vi "Periodic Tasks.vi"() -> ()   [LabVIEW 2014]
doc: "This VI runs in parallel to other tasks. It can contain as many user-defined periodic loops as you need. These can carry out PID or other sorts of timed response."
uses:
  <vilib>/Rock Robotics/WPI/DriverStation/WPI_DriverStationRobotMode2.ctl
  Global Variables.vi
  Robot Global Data.vi
  <vilib>/Utility/file.llb/Read From Spreadsheet File (DBL).vi
  <vilib>/Utility/file.llb/Write To Spreadsheet File (DBL).vi
  <vilib>/addons/control/pid/NI_PID_pid.lvlib
  <vilib>/addons/control/pid/pid.llb/PID (DBL).vi
  NavX Code/navX-MXP Library/navX-MXP IMU.lvlib
  <vilib>/Rock Robotics/WPI/DriverStation/WPI_DriverStationStatusErrorCache.ctl
panel:
  in  "Left Rumble":sgl
  in  "Right Rumble":sgl
  out "Degrees":u16
  out "navX Data":u8[](array[numeric])
  in  "PID gains":T1={"proportional gain (Kc)"=1.0, "integral time (Ti, min)"=0.01, "derivative time (Td, min)"=0.0} {"derivative time (Td, min)" format="%.3f"; "integral time (Ti, min)" format="%.3f"; "proportional gain (Kc)" format="%.3f"}
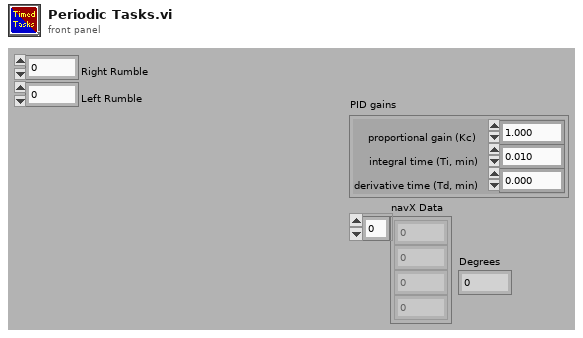
[diagram p1: front panel]
types:
  T1 = cluster{"proportional gain (Kc)":dbl, "integral time (Ti, min)":dbl, "derivative time (Td, min)":dbl}
  T2 = enum16{"Stop", "Three Tote", "Two Tote", "One Tote", "Step", "Top", "Home", "Joystick"}
  T3 = typedef "navX-MXP IMU.lvlib/navX Device TypeDef.ctl" = cluster{"navX Interface Protocol":T4, "navX Interface Protocol TypeDefs":cluster{"SPIDevRef":T5, "I2CDevRef":T8}, "navX System Information":cluster{"Board Information":T10, "Status":T11, "Offsets":T15}, "navX Common Information":cluster{"Update Rate (4Hz-60Hz)":T16, "refnum name":string, "error":errorcluster}}
  T4 = typedef "navX-MXP IMU.lvlib/navX Interface Protocol.ctl" = enum16{"SPI", "I2C"}
  T5 = typedef "WPI_SPIDevRef.ctl" = cluster{"DevStatus":errorcluster, "Handle":i32, "Controller":T6, "SPI Bus":T7}
  T6 = typedef "FPGA_TypedefDigitalModule.ctl" = enum16{"Controller 1"}
  T7 = typedef "spi_bus.ctl" = enum16{"SPI On-Board, CS0", "SPI On-Board, CS1", "SPI On-Board, CS2", "SPI On-Board, CS3", "SPI MXP", "Invalid"}
  T8 = typedef "WPI_I2CDevRef.ctl" = cluster{"DevStatus":errorcluster, "Controller":T6, "Device Address":u8, "Handle":i32, "I2C Bus":T9}
  T9 = typedef "i2c_bus.ctl" = enum16{"I2C On-Board", "I2C MXP", "Invalid"}
  T10 = typedef "navX-MXP IMU.lvlib/navX Board Information.ctl" = cluster{"WhoAmI (50 | 0x32)":u8, "Board Revision":u8, "Firmware Major Version":u8, "Firmware Minor Version":u8}
  T11 = typedef "navX-MXP IMU.lvlib/navX Status Data.ctl" = cluster{"Update Rate Hz":u8, "Accelerometer Full-Scale Range":u8, "Gyro Full-Scale Range":u16, "NAVX_OP_STATUS":T12, "NAVX_CAL_STATUS":T13, "NAVX_SELFTEST_STATUS":u8, "NAVX_SENSOR_STATUS":T14}
  T12 = typedef "navX-MXP IMU.lvlib/navX NAVX_OP_STATUS.ctl" = u8
  T13 = typedef "navX-MXP IMU.lvlib/navX NAVX_CAL_STATUS.ctl" = u8
  T14 = typedef "navX-MXP IMU.lvlib/navX NAVX_SENSOR_STATUS.ctl" = cluster{"MOVING":bool, "YAW_STABLE":bool, "MAG_DISTURBANCE":bool, "ALTITUDE_VALID":bool, "SEALEVEL_PRESS_SET":bool, "FUSED_HEADING_VALID":bool}
  T15 = typedef "navX-MXP IMU.lvlib/navX Offsets Data.ctl" = cluster{"Yaw":dbl, "Quat W":dbl, "Quat X":dbl, "Quat Y":dbl, "Quat Z":dbl}
  T16 = typedef "navX-MXP IMU.lvlib/navX Update Rate.ctl" = u8
  T17 = typedef "WPI_DriverStationStatusErrorCache.ctl" = enum16{"Get", "Set"}
  T18 = typedef "WPI_JoystickDevRef.ctl" = cluster{"Device":T19}
  T19 = typedef "WPI_JoystickDeviceEnum.ctl" = enum16{"USB 0", "USB 1", "USB 2", "USB 3", "USB 4", "USB 5"}
  T20 = typedef "WPI_MotorControlDeviceRef.ctl" = cluster{"DeviceStatus":errorcluster, "Type":T21, "PWM":cluster{"Controller":T6, "PWM Channel":T22, "DeadBand":T23}, "CAN":cluster{"Device Number":u8, "Control Mode":T24, "Semaphore":T25, "Max Vout":dbl, "TalonSRX Control Mode":T26}, "Invert":bool, "TransformRef":T27, "InvTransformRef":T27}
  T21 = typedef "WPI_MotorControlType.ctl" = enum16{"PWM", "CAN", "CANTalonSRX"}
  T22 = typedef "FPGA_DIOPWMChannel.ctl" = enum8{"PWM 0", "PWM 1", "PWM 2", "PWM 3", "PWM 4", "PWM 5", "PWM 6", "PWM 7", "PWM 8", "PWM 9", "PWM MXP 0", "PWM MXP 1", "PWM MXP 2", "PWM MXP 3", "PWM MXP 4", "PWM MXP 5", "PWM MXP 6", "PWM MXP 7", "PWM MXP 8", "PWM MXP 9", "Invalid"}
  T23 = typedef "WPI_PWMDeadband.ctl" = cluster{"Name":string, "maxPositivePwm":i32, "minPositivePwm":i32, "centerPwm":i32, "maxNegativePwm":i32, "minNegativePwm":i32, "angularRange":u16}
  T24 = typedef "WPI_CANJaguar_ControlMode.ctl" = enum8{"Percent VBus", "Current", "Speed", "Position", "Voltage"}
  T25 = typedef "Semaphore RefNum" = refnum<k1>
  T26 = typedef "WPI_CANTalonSRX_APIControlMode.ctl" = enum8{"Percent VBus", "Speed", "Position", "Slave", "Unchanged / Invalid"}
  T27 = typedef "WPI_PWMTransform_ConPane.ctl" = refnum<vi>
  T28 = typedef "WPI_DriverStationRobotMode2.ctl" = enum16{"Autonomous Disabled", "Autonomous Enabled", "Teleop Disabled", "Teleop Enabled", "Disconnected", "Finish", "Test Disabled", "Test Enabled", "Emergency Stopped"}
  T29 = typedef "WPI_CounterDevRef.ctl" = cluster{"DevStatus":errorcluster, "CntIndex":T30}
  T30 = typedef "FPGA_CounterCtrSystemIndex.ctl" = enum8{"Ctr 0", "Ctr 1", "Ctr 2", "Ctr 3", "Ctr 4", "Ctr 5", "Ctr 6", "Ctr 7", "Invalid"}
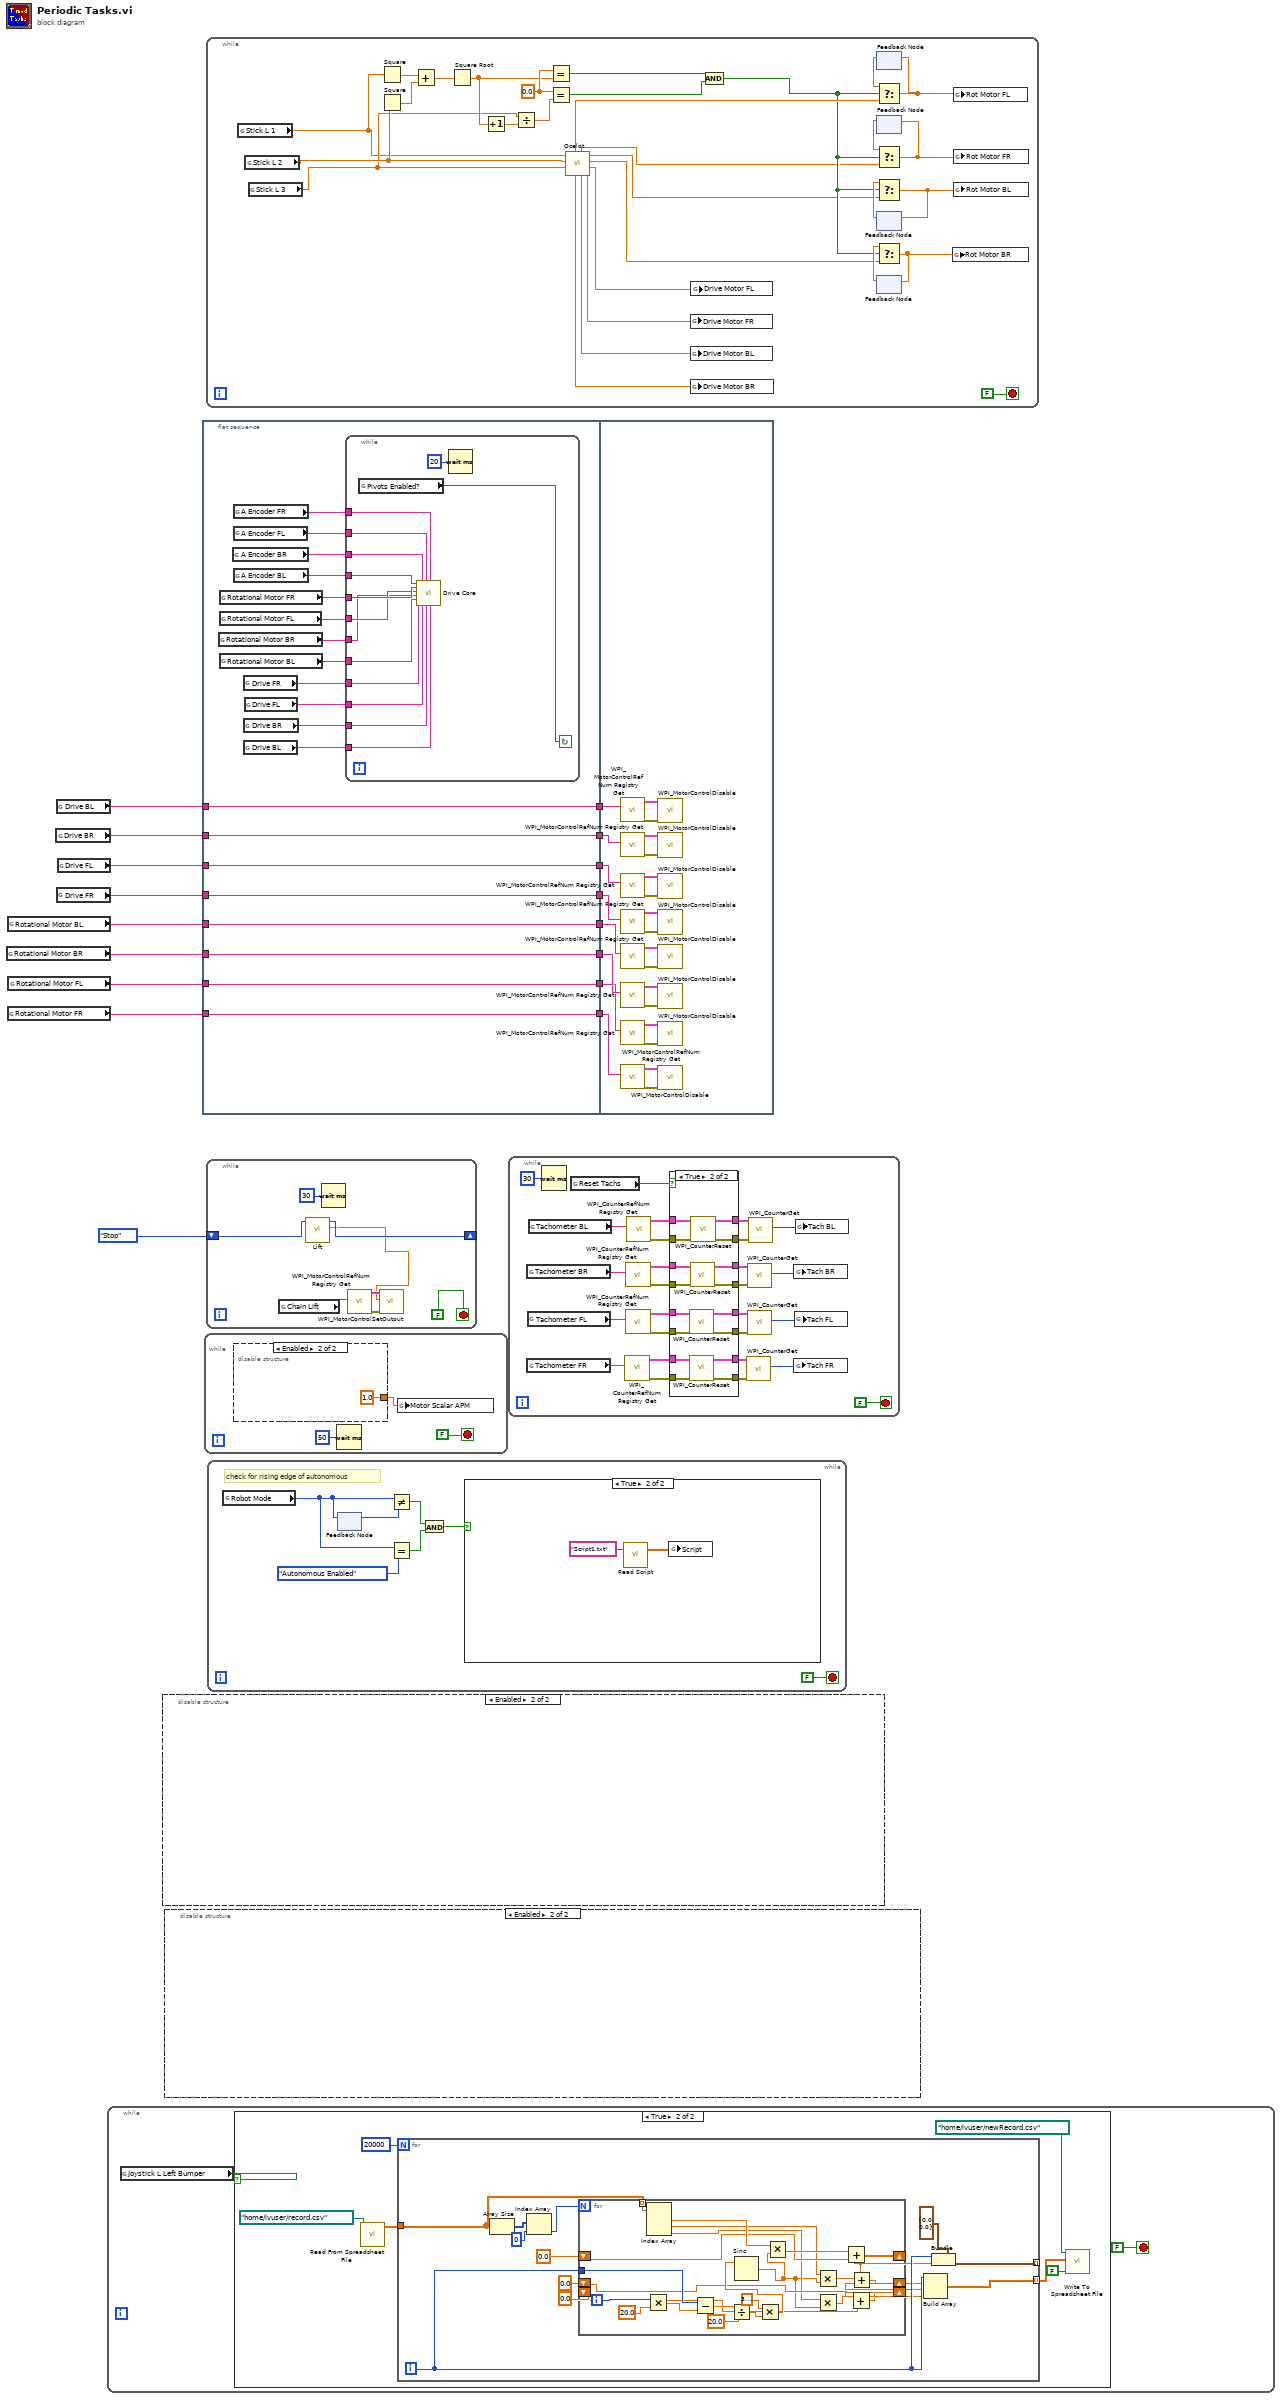
[diagram p0: block diagram]
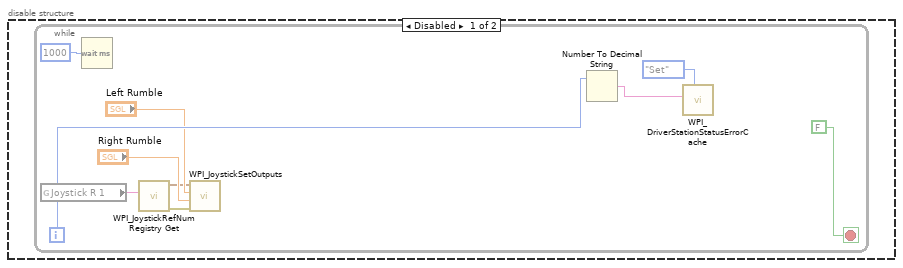
[diagram p3: hidden frame]
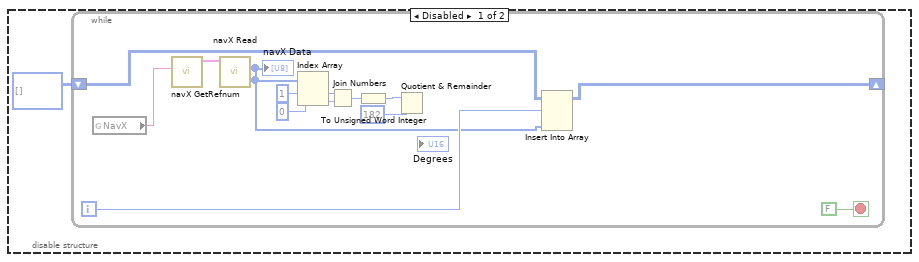
[diagram p4: hidden frame]
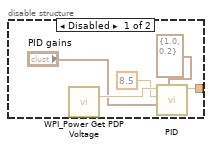
[diagram p7: hidden frame]
diagram:
  n1 = global read "Global Variables.vi" "Rotational Motor BR"() -> (w6:string)
  n2 = global read "Global Variables.vi" "Rotational Motor BL"() -> (w8:string)
  n3 = global read "Global Variables.vi" "Rotational Motor FR"() -> (w2:string)
  n4 = global read "Global Variables.vi" "Rotational Motor FL"() -> (w4:string)
  n5 = global read "Global Variables.vi" "Drive BR"() -> (w14:string)
  n6 = global read "Global Variables.vi" "Drive BL"() -> (w16:string)
  n7 = global read "Global Variables.vi" "Drive FR"() -> (w10:string)
  n8 = global read "Global Variables.vi" "Drive FL"() -> (w12:string)
  n9 = while {
    stop <- FALSE stop-if-true
    n10 = global read "Global Variables.vi" "Joystick L Left Bumper"() -> (w18:bool)
    n11 = case shown="True" w18 {
      frame False {
      }
      frame True {
        n12 = call-poly <vilib>:"Read From Spreadsheet File.vi"("file path (dialog if empty)"=path "/home/lvuser/record.csv") -> ("all rows"=w24:dbl[][])  [unwired: 6 in, 4 out]
        n13 = for {
          N: 20000 -> [_]
          tunnel: [w34] -> _ mode=indexing
          tunnel: w24 -> [w33]
          tunnel: [w30] -> w23 mode=indexing
          i -> [w32]
          n14 = Array Size(array=w33) -> (size(s)=w39:i32[])
          n15 = Index Array(array=w39, index=0) -> (element=w38:i32)
          n16 = for {
            N: w38 -> [_]
            shift-right: [w49] -> w31
            shift-left: 0.0 -> [w51]
            tunnel: w33 -> [w60] mode=indexing
            tunnel: w32 -> [w52]
            shift-right: [w47] -> w29
            shift-left: 0.0 -> [w44]
            shift-right: [w48] -> w28
            shift-left: 0.0 -> [w43]
            i -> [w58]
            n17 = Multiply(x=w58, y=20.0) -> (x*y=w55:dbl)
            n18 = Index Array(array=w60) -> (element #1=w61:dbl, element #2=w42:dbl, element #3=w41:dbl)  [unwired: 3 in]
            n19 = Subtract(x=w52, y=w55) -> (x-y=w57:dbl)
            n20 = Divide(x=w57, y=20.0) -> (x/y=w54:dbl)
            n21 = Multiply(x=3.141592653589793, y=w54) -> (x*y=w50:dbl)
            n22 = Sinc(1:w50) -> (0:w40:dbl)
            n23 = Multiply(x=w61, y=w40) -> (x*y=w62:dbl)
            n24 = Multiply(x=w42, y=w40) -> (x*y=w45:dbl)
            n25 = Multiply(x=w41, y=w40) -> (x*y=w46:dbl)
            n26 = Add(x=w62, y=w51) -> (x+y=w49:dbl)
            n27 = Add(x=w46, y=w43) -> (x+y=w48:dbl)
            n28 = Add(x=w45, y=w44) -> (x+y=w47:dbl)
          }
          n29 = Build Array(w32, w31, w29, w28) -> (w30:dbl[])
          n30 = Bundle(cluster=cluster{dbl, dbl} {0.0, 0.0}, w32, w31) -> (w34:cluster{dbl, dbl})
        }
        n31 = call-poly <vilib>:"Write To Spreadsheet File.vi"("append to file? (new file:F)"=FALSE, "2D data"=w23, "file path (dialog if empty)"=path "/home/lvuser/newRecord.csv") -> ()  [unwired: 5 in, 1 out]
      }
    }
  }
  n32 = disable-structure shown="Enabled" {
    frame Disabled {
      n33 = while {
        shift-right: [w66] -> _
        shift-left: u16[][] [] -> [w65]
        i -> [w67]
        stop <- FALSE stop-if-true
        n34 = global read "Global Variables.vi" "NavX"() -> (w75:string)
        n35 = call "navX GetRefnum.vi"("refnum name"=w75) -> ("navX Device TypeDef"=w76:T3)  [unwired: 9 in, 1 out]
        n36 = call "navX Read.vi"("navX Device TypeDef"=w76) -> ("navX Data"=w64:u8[])  [unwired: 8 in, 2 out]
        "navX Data" <- w64
        n37 = Index Array(array=w64, index #1=1 ("index"), index #2=0 ("index")) -> (element #1=w74:u8, element #2=w73:u8)
        n38 = Join Numbers(hi=w74, lo=w73) -> ((hi.lo)=w70:u16)
        n39 = To Unsigned Word Integer(number=w70) -> (unsigned 16bit integer=w69:u16)
        n40 = Quotient & Remainder(x=w69, y=u16 182) -> ()  [unwired: 2 out]
        n41 = Insert Into Array(array=w65, index (row)=w67, new element=w64) -> (w66:u16[][])  [unwired: 1 in]
      }
    }
    frame Enabled {
    }
  }
  n42 = disable-structure shown="Enabled" {
    frame Disabled {
      n43 = while {
        i -> [w84]
        stop <- FALSE stop-if-true
        n44 = global read "Global Variables.vi" "Joystick R 1"() -> (w79:string)
        n45 = Wait (ms)(milliseconds to wait=u32 1000) -> ()  [unwired: 1 out]
        n46 = call <vilib>:"WPI_JoystickRefNum Registry Get.vi"("refnum name"=w79) -> ("error out"=w78:errorcluster, "JoystickDevRef"=w80:T18)  [unwired: 9 in]
        n47 = call <vilib>:"WPI_JoystickSetOutputs.vi"("error in (no error)"=w78, "Right Rumble"="Right Rumble", "Left Rumble"="Left Rumble", "JoystickDevRef"=w80) -> ()  [unwired: 6 in, 2 out]
        n48 = Number To Decimal String(number=w84) -> (decimal integer string=w85:string)  [unwired: 1 in]
        n49 = call <vilib>:"WPI_DriverStationStatusErrorCache.vi"("StatusErrorCacheOp"=WPI_DriverStationStatusErrorCache."Set", "Error String"=w85) -> ()  [unwired: 1 in, 9 out]
      }
    }
    frame Enabled {
    }
  }
  n50 = flat-sequence {
    tunnel: [w95] -> w17
    tunnel: w16 -> [w95]
    tunnel: [w94] -> w15
    tunnel: w14 -> [w94]
    tunnel: [w93] -> w13
    tunnel: w12 -> [w93]
    tunnel: [w92] -> w11
    tunnel: w10 -> [w92]
    tunnel: [w91] -> w9
    tunnel: w8 -> [w91]
    tunnel: [w90] -> w7
    tunnel: w6 -> [w90]
    tunnel: [w89] -> w5
    tunnel: w4 -> [w89]
    tunnel: [w88] -> w3
    tunnel: w2 -> [w88]
    tunnel: w17 -> [w129]
    tunnel: w15 -> [w128]
    tunnel: w13 -> [w127]
    tunnel: w11 -> [w126]
    tunnel: w9 -> [w125]
    tunnel: w7 -> [w124]
    tunnel: w5 -> [w123]
    tunnel: w3 -> [w122]
    frame #0 {
      n51 = global read "Global Variables.vi" "Rotational Motor BR"() -> (w101:string)
      n52 = global read "Global Variables.vi" "Rotational Motor FR"() -> (w103:string)
      n53 = global read "Global Variables.vi" "Rotational Motor FL"() -> (w102:string)
      n54 = global read "Global Variables.vi" "Rotational Motor BL"() -> (w100:string)
      n55 = global read "Global Variables.vi" "A Encoder BR"() -> (w105:string)
      n56 = global read "Global Variables.vi" "A Encoder FR"() -> (w107:string)
      n57 = global read "Global Variables.vi" "A Encoder FL"() -> (w106:string)
      n58 = global read "Global Variables.vi" "A Encoder BL"() -> (w104:string)
      n59 = global read "Global Variables.vi" "Drive FR"() -> (w99:string)
      n60 = global read "Global Variables.vi" "Drive BR"() -> (w97:string)
      n61 = global read "Global Variables.vi" "Drive BL"() -> (w96:string)
      n62 = global read "Global Variables.vi" "Drive FL"() -> (w98:string)
      n63 = while {
        tunnel: w107 -> [w120]
        tunnel: w106 -> [w119]
        tunnel: w105 -> [w118]
        tunnel: w104 -> [w117]
        tunnel: w103 -> [w116]
        tunnel: w102 -> [w115]
        tunnel: w101 -> [w114]
        tunnel: w100 -> [w113]
        tunnel: w99 -> [w112]
        tunnel: w98 -> [w111]
        tunnel: w97 -> [w110]
        tunnel: w96 -> [w109]
        stop <- w121 continue-if-true
        n64 = global read "Global Variables.vi" "Pivots Enabled?"() -> (w121:bool)
        n65 = call "Drive Core.vi"("A Encoder BL"=w117, "Rotational Motor FR"=w116, "Rotational Motor FL"=w115, "Rotational Motor BR"=w114, "Rotational Motor BL"=w113, "Drive Motor FR"=w112, "A Encoder BR"=w118, "Drive Motor FL"=w111, "A Encoder FL"=w119, "Drive Motor BR"=w110, "A Encoder FR"=w120, "Drive Motor BL"=w109) -> ()  [unwired: 8 in]
        n66 = Wait (ms)(milliseconds to wait=u32 20) -> ()  [unwired: 1 out]
      }
    }
    frame #1 {
      n67 = call <vilib>:"WPI_MotorControlRefNum Registry Get.vi"("refnum name"=w129) -> ("error out"=w145:errorcluster, "MotorControlDevRef"=w144:T20)  [unwired: 9 in]
      n68 = call <vilib>:"WPI_MotorControlRefNum Registry Get.vi"("refnum name"=w128) -> ("error out"=w143:errorcluster, "MotorControlDevRef"=w142:T20)  [unwired: 9 in]
      n69 = call <vilib>:"WPI_MotorControlRefNum Registry Get.vi"("refnum name"=w127) -> ("error out"=w141:errorcluster, "MotorControlDevRef"=w140:T20)  [unwired: 9 in]
      n70 = call <vilib>:"WPI_MotorControlRefNum Registry Get.vi"("refnum name"=w126) -> ("error out"=w139:errorcluster, "MotorControlDevRef"=w138:T20)  [unwired: 9 in]
      n71 = call <vilib>:"WPI_MotorControlRefNum Registry Get.vi"("refnum name"=w125) -> ("error out"=w137:errorcluster, "MotorControlDevRef"=w136:T20)  [unwired: 9 in]
      n72 = call <vilib>:"WPI_MotorControlRefNum Registry Get.vi"("refnum name"=w124) -> ("error out"=w135:errorcluster, "MotorControlDevRef"=w134:T20)  [unwired: 9 in]
      n73 = call <vilib>:"WPI_MotorControlRefNum Registry Get.vi"("refnum name"=w123) -> ("error out"=w133:errorcluster, "MotorControlDevRef"=w132:T20)  [unwired: 9 in]
      n74 = call <vilib>:"WPI_MotorControlRefNum Registry Get.vi"("refnum name"=w122) -> ("error out"=w131:errorcluster, "MotorControlDevRef"=w130:T20)  [unwired: 9 in]
      n75 = call <vilib>:"WPI_MotorControlDisable.vi"("error in (no error)"=w145, "MotorControlDevRef"=w144) -> ()  [unwired: 8 in, 2 out]
      n76 = call <vilib>:"WPI_MotorControlDisable.vi"("error in (no error)"=w143, "MotorControlDevRef"=w142) -> ()  [unwired: 8 in, 2 out]
      n77 = call <vilib>:"WPI_MotorControlDisable.vi"("error in (no error)"=w141, "MotorControlDevRef"=w140) -> ()  [unwired: 8 in, 2 out]
      n78 = call <vilib>:"WPI_MotorControlDisable.vi"("error in (no error)"=w139, "MotorControlDevRef"=w138) -> ()  [unwired: 8 in, 2 out]
      n79 = call <vilib>:"WPI_MotorControlDisable.vi"("error in (no error)"=w137, "MotorControlDevRef"=w136) -> ()  [unwired: 8 in, 2 out]
      n80 = call <vilib>:"WPI_MotorControlDisable.vi"("error in (no error)"=w135, "MotorControlDevRef"=w134) -> ()  [unwired: 8 in, 2 out]
      n81 = call <vilib>:"WPI_MotorControlDisable.vi"("error in (no error)"=w133, "MotorControlDevRef"=w132) -> ()  [unwired: 8 in, 2 out]
      n82 = call <vilib>:"WPI_MotorControlDisable.vi"("error in (no error)"=w131, "MotorControlDevRef"=w130) -> ()  [unwired: 8 in, 2 out]
    }
  }
  n83 = while {
    stop <- FALSE stop-if-true
    n84 = disable-structure shown="Enabled" {
      disable-tunnel: [w149 1.0 ("Motor Scalar APM")] -> w146
      frame Disabled {
        n85 = call <vilib>:"WPI_Power Get PDP Voltage.vi"() -> ("voltage (V)"=w152:dbl)  [unwired: 14 in, 1 out]
        n86 = call-poly <vilib>:"PID.vi"("output range"=cluster{"output high":dbl, "output low":dbl} {"output high"=1.0, "output low"=0.2}, "PID gains"="PID gains", "process variable"=8.5 ("setpoint"), "setpoint"=w152) -> ("output"=w149:dbl)  [unwired: 6 in, 1 out]
      }
      frame Enabled {
      }
    }
    n87 = Wait (ms)(milliseconds to wait=u32 50) -> ()  [unwired: 1 out]
    n88 = global write "Global Variables.vi" "Motor Scalar APM"(w146) -> ()
  }
  n89 = while {
    stop <- FALSE stop-if-true
    w181 = 0.0 ("x")
    n90 = global read "Global Variables.vi" "Stick L 1"() -> (w156:dbl)
    n91 = global read "Global Variables.vi" "Stick L 2"() -> (w158:dbl)
    n92 = global read "Global Variables.vi" "Stick L 3"() -> (w157:dbl)
    n93 = Square(x=w156) -> (x^2=w183:dbl)
    n94 = Square(x=w158) -> (x^2=w184:dbl)
    n95 = Add(x=w183, y=w184) -> (x+y=w182:dbl)
    n96 = Square Root(x=w182) -> (sqrt(x)=w180:dbl)
    n97 = Increment(x=w180) -> (x+1=w179:dbl)
    n98 = Divide(x=w157, y=w179) -> (x/y=w178:dbl)
    n99 = Equal?(x=w181, y=w180) -> (x = y?=w172:bool)
    n100 = Equal?(x=w181, y=w178) -> (x = y?=w171:bool)
    n101 = call "Ocelot.vi"("RCW (X2)"=w157, "FWD (Y)"=w158, "STR (X)"=w156) -> ("FRD"=w161:dbl, "FLD"=w162:dbl, "BRS"=w163:dbl, "BLS"=w164:dbl, "BLD"=w160:dbl, "FRS"=w165:dbl, "BRD"=w159:dbl, "FLS"=w173:dbl)  [unwired: 1 in]
    n102 = global write "Global Variables.vi" "Drive Motor FR"(w161) -> ()
    n103 = global write "Global Variables.vi" "Drive Motor BL"(w160) -> ()
    n104 = global write "Global Variables.vi" "Drive Motor BR"(w159) -> ()
    n105 = global write "Global Variables.vi" "Drive Motor FL"(w162) -> ()
    n106 = And(x=w172, y=w171) -> (x .and. y?=w170:bool)
    n107 = feedback #1() -> (w177:dbl)  [unwired: 1 in]
    n108 = Select(t=w177, s=w170, f=w173) -> (s? t:f=w169:dbl)
    n109 = feedback-in #1(w169) -> ()
    n110 = feedback #2() -> (w176:dbl)  [unwired: 1 in]
    n111 = Select(t=w176, s=w170, f=w165) -> (s? t:f=w168:dbl)
    n112 = feedback-in #2(w168) -> ()
    n113 = feedback #3() -> (w175:dbl)  [unwired: 1 in]
    n114 = Select(t=w175, s=w170, f=w164) -> (s? t:f=w167:dbl)
    n115 = feedback-in #3(w167) -> ()
    n116 = feedback #4() -> (w174:dbl)  [unwired: 1 in]
    n117 = Select(t=w174, s=w170, f=w163) -> (s? t:f=w166:dbl)
    n118 = feedback-in #4(w166) -> ()
    n119 = global write "Global Variables.vi" "Rot Motor BR"(w166) -> ()
    n120 = global write "Global Variables.vi" "Rot Motor FL"(w169) -> ()
    n121 = global write "Global Variables.vi" "Rot Motor FR"(w168) -> ()
    n122 = global write "Global Variables.vi" "Rot Motor BL"(w167) -> ()
  }
  n123 = while {
    shift-right: [w190] -> _
    shift-left: T2."Stop" ("State Out") -> [w191]
    stop <- FALSE stop-if-true
    n124 = global read "Global Variables.vi" "Chain Lift"() -> (w185:string)
    n125 = call "Lift.vi"("State"=w191) -> ("Lift Motor(Global...)"=w186:dbl, "State Out"=w190:T2)  [unwired: 9 in]
    n126 = Wait (ms)(milliseconds to wait=u32 30) -> ()  [unwired: 1 out]
    n127 = call <vilib>:"WPI_MotorControlRefNum Registry Get.vi"("refnum name"=w185) -> ("error out"=w189:errorcluster, "MotorControlDevRef"=w188:T20)  [unwired: 9 in]
    n128 = call <vilib>:"WPI_MotorControlSetOutput.vi"("error in (no error)"=w189, "Output"=w186, "MotorControlDevRef"=w188) -> ()  [unwired: 6 in, 3 out]
  }
  n129 = while {
    stop <- FALSE stop-if-true
    # "check for rising edge of autonomous"
    n130 = global read "Robot Global Data.vi" "Robot Mode"() -> (w197:T28)
    n131 = feedback #5() -> (w199:T28)  [unwired: 1 in]
    n132 = feedback-in #5(w197) -> ()
    n133 = Not Equal?(x=w197, y=w199) -> (x != y?=w195:bool)
    n134 = Equal?(x=w197, y=WPI_DriverStationRobotMode2."Autonomous Enabled" ("Robot Mode")) -> (x = y?=w196:bool)
    n135 = And(x=w195, y=w196) -> (x .and. y?=w193:bool)
    n136 = case shown="True" w193 {
      frame False {
      }
      frame True {
        n137 = call "Read Script.vi"("script name"="Script1.txt") -> ("output array"=w200:dbl[][])  [unwired: 1 in, 1 out]
        n138 = global write "Global Variables.vi" "Script"(w200) -> ()
      }
    }
  }
  n139 = while {
    stop <- FALSE stop-if-true
    n140 = global read "Global Variables.vi" "Tachometer BR"() -> (w215:string)
    n141 = global read "Global Variables.vi" "Tachometer FR"() -> (w203:string)
    n142 = global read "Global Variables.vi" "Tachometer FL"() -> (w214:string)
    n143 = global read "Global Variables.vi" "Tachometer BL"() -> (w227:string)
    n144 = Wait (ms)(milliseconds to wait=u32 30) -> ()  [unwired: 1 out]
    n145 = global read "Global Variables.vi" "Reset Tachs"() -> (w226:bool)
    n146 = call <vilib>:"WPI_CounterRefNum Registry Get.vi"("refnum name"=w203) -> ("error out"=w205:errorcluster, "CounterDevRef"=w204:T29)  [unwired: 9 in]
    n147 = call <vilib>:"WPI_CounterRefNum Registry Get.vi"("refnum name"=w215) -> ("error out"=w217:errorcluster, "CounterDevRef"=w216:T29)  [unwired: 9 in]
    n148 = call <vilib>:"WPI_CounterRefNum Registry Get.vi"("refnum name"=w214) -> ("error out"=w212:errorcluster, "CounterDevRef"=w213:T29)  [unwired: 9 in]
    n149 = call <vilib>:"WPI_CounterRefNum Registry Get.vi"("refnum name"=w227) -> ("error out"=w224:errorcluster, "CounterDevRef"=w225:T29)  [unwired: 9 in]
    n150 = case shown="True" w226 {
      tunnel: w225 -> [w236 w252]
      tunnel: w224 -> [w235 w251]
      tunnel: [w236 w250] -> w223
      tunnel: [w235 w249] -> w222
      tunnel: w216 -> [w233 w239]
      tunnel: w217 -> [w234 w248]
      tunnel: [w233 w238] -> w218
      tunnel: [w234 w237] -> w219
      tunnel: w213 -> [w232 w240]
      tunnel: w212 -> [w231 w247]
      tunnel: [w232 w241] -> w211
      tunnel: [w231 w242] -> w210
      tunnel: w204 -> [w229 w245]
      tunnel: w205 -> [w230 w246]
      tunnel: [w229 w244] -> w206
      tunnel: [w230 w243] -> w207
      frame False {
      }
      frame True {
        n151 = call <vilib>:"WPI_CounterReset.vi"("error in (no error)"=w247, "CounterDevRef in"=w240) -> ("error out"=w242:errorcluster, "CounterDevRef out"=w241:T29)  [unwired: 8 in]
        n152 = call <vilib>:"WPI_CounterReset.vi"("error in (no error)"=w246, "CounterDevRef in"=w245) -> ("error out"=w243:errorcluster, "CounterDevRef out"=w244:T29)  [unwired: 8 in]
        n153 = call <vilib>:"WPI_CounterReset.vi"("error in (no error)"=w248, "CounterDevRef in"=w239) -> ("error out"=w237:errorcluster, "CounterDevRef out"=w238:T29)  [unwired: 8 in]
        n154 = call <vilib>:"WPI_CounterReset.vi"("error in (no error)"=w251, "CounterDevRef in"=w252) -> ("error out"=w249:errorcluster, "CounterDevRef out"=w250:T29)  [unwired: 8 in]
      }
    }
    n155 = call <vilib>:"WPI_CounterGet.vi"("error in (no error)"=w207, "CounterDevRef in"=w206) -> ("Value"=w208:i32)  [unwired: 4 in, 5 out]
    n156 = call <vilib>:"WPI_CounterGet.vi"("error in (no error)"=w219, "CounterDevRef in"=w218) -> ("Value"=w220:i32)  [unwired: 4 in, 5 out]
    n157 = call <vilib>:"WPI_CounterGet.vi"("error in (no error)"=w210, "CounterDevRef in"=w211) -> ("Value"=w209:i32)  [unwired: 4 in, 5 out]
    n158 = call <vilib>:"WPI_CounterGet.vi"("error in (no error)"=w222, "CounterDevRef in"=w223) -> ("Value"=w221:i32)  [unwired: 4 in, 5 out]
    n159 = global write "Global Variables.vi" "Tach BR"(w220) -> ()
    n160 = global write "Global Variables.vi" "Tach FR"(w208) -> ()
    n161 = global write "Global Variables.vi" "Tach FL"(w209) -> ()
    n162 = global write "Global Variables.vi" "Tach BL"(w221) -> ()
  }
